vi "Main Engine Write Data Log File.vi"(8 "error in":errorcluster, 9 "State":string, 10 "Input Data":string, 11 "Log file path In":path) -> (0 "error out":errorcluster, 3 "Log File Path Out":path)   [LabVIEW 2024]
doc: "All Rights Reserved © 2023 SyncSols"
uses:
  Controls/Main Engine Error Log Cluster.ctl
  Controls/Main Engine Q Option.ctl
  <vilib>/Utility/error.llb/DialogType.ctl
  907b42ce-c0d4-4bed-95ac-a7db4d020177.vi
  <vilib>/JDP Science/JSONtext/Variant to JSON Text.vi
  <vilib>/JDP Science/JSONtext/LVClass Serializer/JSONtext LVClass Serializer.lvclass
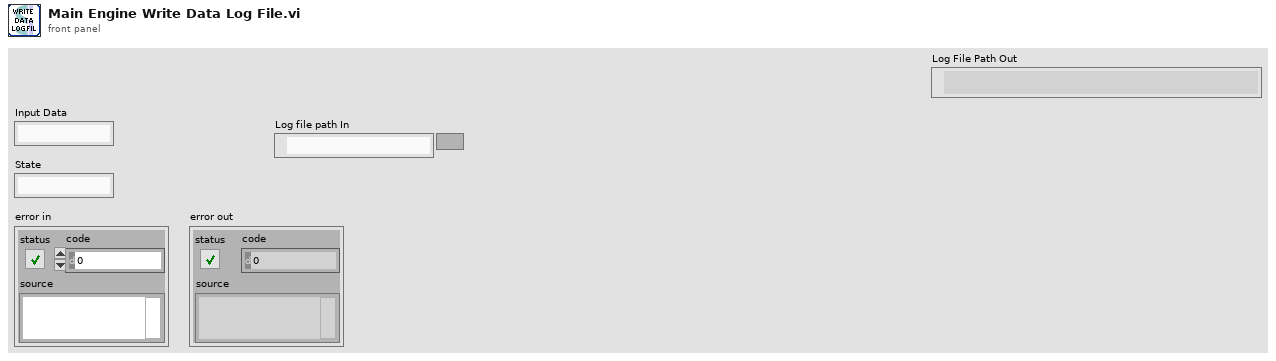
[diagram p1: front panel]
types:
  T1 = enum16{"open", "replace", "create", "open or create", "replace or create", "replace or create with confirmation"}
  T2 = typedef "Main Engine Error Log Cluster.ctl" = cluster{"Interface":string, "Interface Data":cluster{"Command":string, "SubCmd":string, "Data":string}}
  T3 = typedef "Main Engine Q Option.ctl" = enum16{"Init", "Get"}
  T4 = typedef "DialogType.ctl" = u16
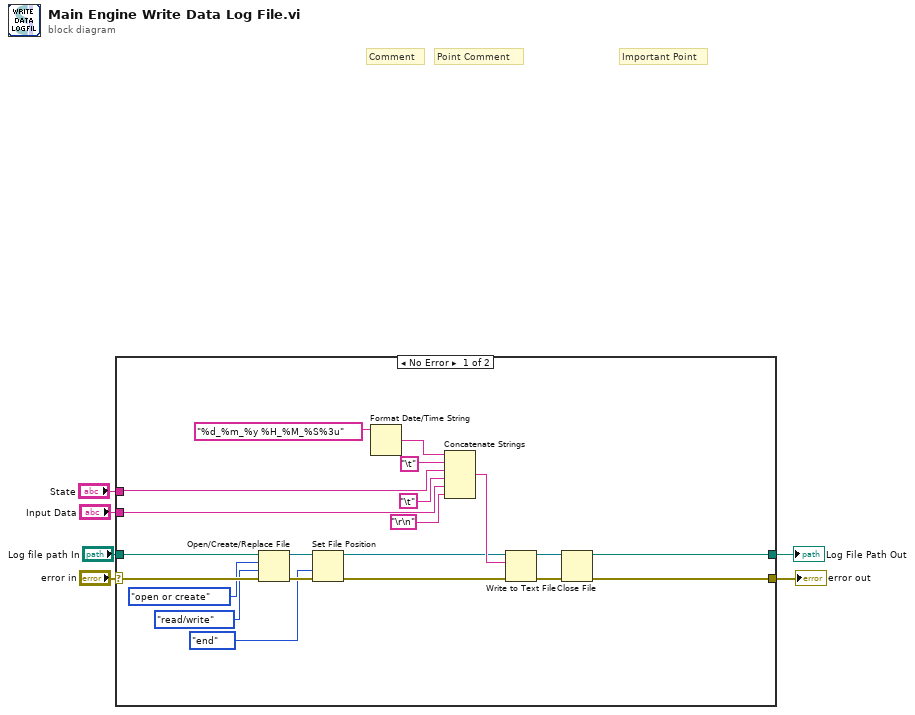
[diagram p0: block diagram]
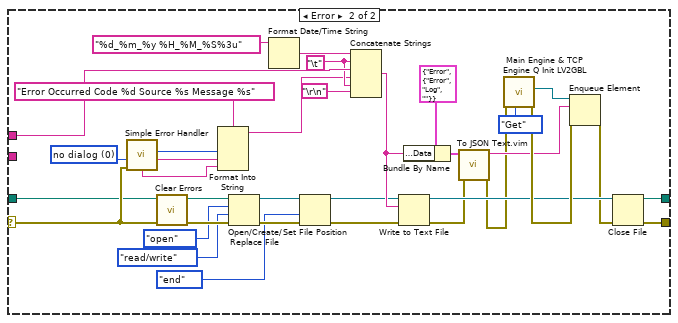
[diagram p2: hidden frame]
diagram:
  # "Important Point"
  # "Point Comment"
  # "Comment"
  n1 = case shown="No Error" "error in" {
    selector: "error in" -> [w15 w54]
    tunnel: [w17 w38] -> w6
    tunnel: "Input Data" -> [w27 _]
    tunnel: "State" -> [w22 w58]
    tunnel: "Log file path In" -> [w14 w44]
    tunnel: [w16 w37] -> w1
    frame No Error {
      n2 = Open/Create/Replace File(file path (use dialog)=w14, error in=w15, operation (0:open)=T1."open or create", access (0:read/write)=enum16{"read/write", "read-only", "write-only"}."read/write") -> (refnum out=w11:refnum<file>, error out=w9:errorcluster)  [unwired: 2 in, 1 out]
      n3 = Set File Position(refnum=w11, from (0:start)=enum16{"start", "end", "current"}."end", error in=w9) -> (refnum out=w10:refnum<file>, error out=w8:errorcluster)  [unwired: 1 in]
      n4 = Format Date/Time String(time format string (%c)="%d_%m_%y %H_%M_%S%3u") -> (date/time string=w20:string)  [unwired: 2 in]
      n5 = Concatenate Strings(w20, "\t", w22, "\t", w27, "\r\n") -> (w23:string)
      n6 = Write to Text File(file (use dialog)=w10, text=w23, error in=w8) -> (refnum out=w19:refnum<file>, error out=w18:errorcluster)  [unwired: 1 in, 1 out]
      n7 = Close File(refnum=w19, error in=w18) -> (path=w16:path, error out=w17:errorcluster)
    }
    frame Error {
      w53 = T4 0 items=["no dialog", "OK message", "continue or stop message", "OK message + warnings", "continue/stop + warnings"] ("type of dialog (OK msg:1)")
      w56 = "\t"
      n8 = call <vilib>:"Simple Error Handler.vi"("type of dialog (OK msg:1)"=w53, "error in (no error)"=w54) -> ("code out"=w52:i32, "source out"=w51:string, "message"=w50:string)  [unwired: 3 in, 2 out]
      n9 = call <vilib>:"Clear Errors.vi"("error in (no error)"=w54) -> ("error out"=w43:errorcluster)  [unwired: 5 in, 1 out]
      n10 = Format Into String "Format Into String"(format string="Error Occurred Code %d Source %s Message %s" ("string"), w52, w51, w50) -> (resulting string=w55:string)  [unwired: 2 in, 1 out]
      n11 = Open/Create/Replace File(file path (use dialog)=w44, error in=w43, operation (0:open)=T1."open", access (0:read/write)=enum16{"read/write", "read-only", "write-only"}."read/write") -> (refnum out=w32:refnum<file>, error out=w31:errorcluster)  [unwired: 2 in, 1 out]
      n12 = Format Date/Time String(time format string (%c)="%d_%m_%y %H_%M_%S%3u") -> (date/time string=w59:string)  [unwired: 2 in]
      n13 = Set File Position(refnum=w32, from (0:start)=enum16{"start", "end", "current"}."end", error in=w31) -> (refnum out=w30:refnum<file>, error out=w29:errorcluster)  [unwired: 1 in]
      n14 = Concatenate Strings(w59, w56, w58, w55, w56, "\r\n") -> (w45:string)
      n15 = Write to Text File(file (use dialog)=w30, text=w45, error in=w29) -> (refnum out=w40:refnum<file>, error out=w35:errorcluster)  [unwired: 1 in, 1 out]
      n16 = Bundle By Name(cluster=T2 {"Interface"="Error", "Interface Data"={"Command"="Error", "SubCmd"="Log", "Data"=""}}, "Interface Data.Data"=w45) -> (w36:T2)
      n17 = call "To JSON Text.vim"("error in (no error)"=w35, "Anything"=w36) -> ("error out"=w33:errorcluster, "<JSON>"=w34:string)  [unwired: 8 in]
      n18 = call "Main Engine & TCP Engine Q Init LV2GBL.vi"("Q Option"=Main_Engine_Q_Option."Get", "error in"=w33) -> ("error out"=w48:errorcluster, "TCP Enigine Tx-Q"=w47:refnum<queue>)  [unwired: 7 in, 1 out]
      n19 = Enqueue Element(queue=w47, element=w34, error in (no error)=w48) -> (error out=w39:errorcluster)  [unwired: 1 in, 2 out]
      n20 = Close File(refnum=w40, error in=w39) -> (path=w37:path, error out=w38:errorcluster)
    }
  }
  "error out" <- w6
  "Log File Path Out" <- w1
